vi "Turn To Angle Teleop.vi"(8 "Z Axis":dbl, 9 "PID gains":T1={"proportional gain (Kc)"=0.035, "integral time (Ti, min)"=0.0, "derivative time (Td, min)"=0.0018}, 10 "POV":i16(knob) scale=0.0..360.0, 11 "output range":cluster{"output high":dbl, "output low":dbl}={"output high"=1.0, "output low"=-1.0}) -> (2 "Adjustment Voltage":dbl)   [LabVIEW 2018]
uses:
  <vilib>/addons/control/pid/pid.llb/PID (DBL).vi
  <vilib>/addons/control/pid/NI_PID_pid.lvlib
panel:
  # ".0202"
  # "0"
  # ".0032150"
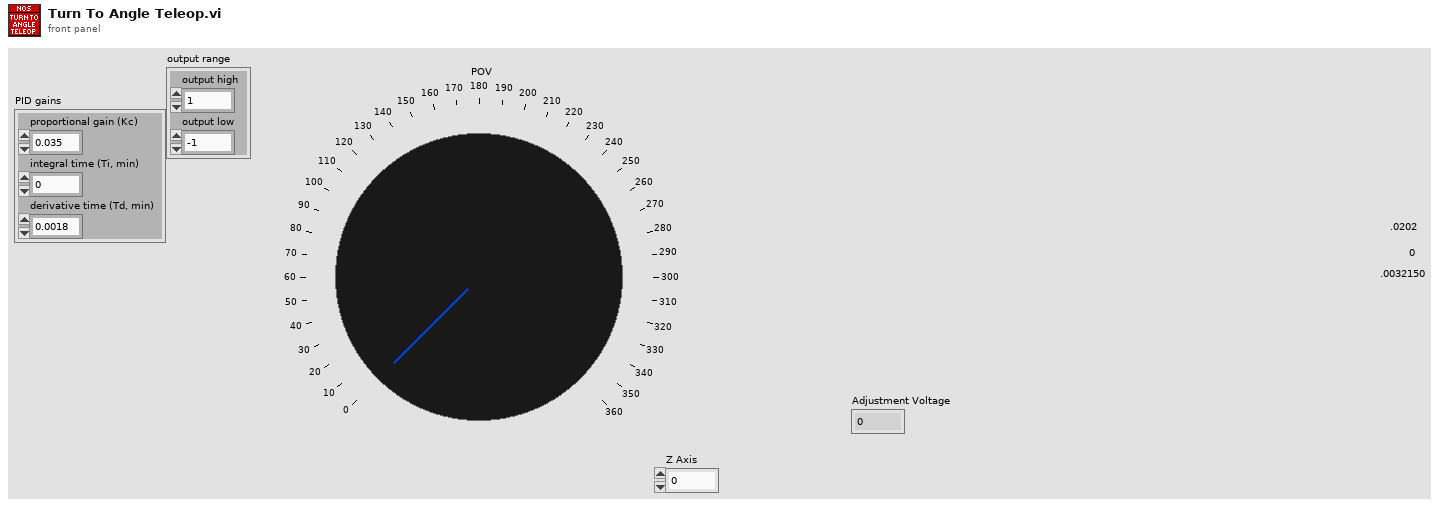
[diagram p1: front panel]
types:
  T1 = cluster{"proportional gain (Kc)":dbl, "integral time (Ti, min)":dbl, "derivative time (Td, min)":dbl}
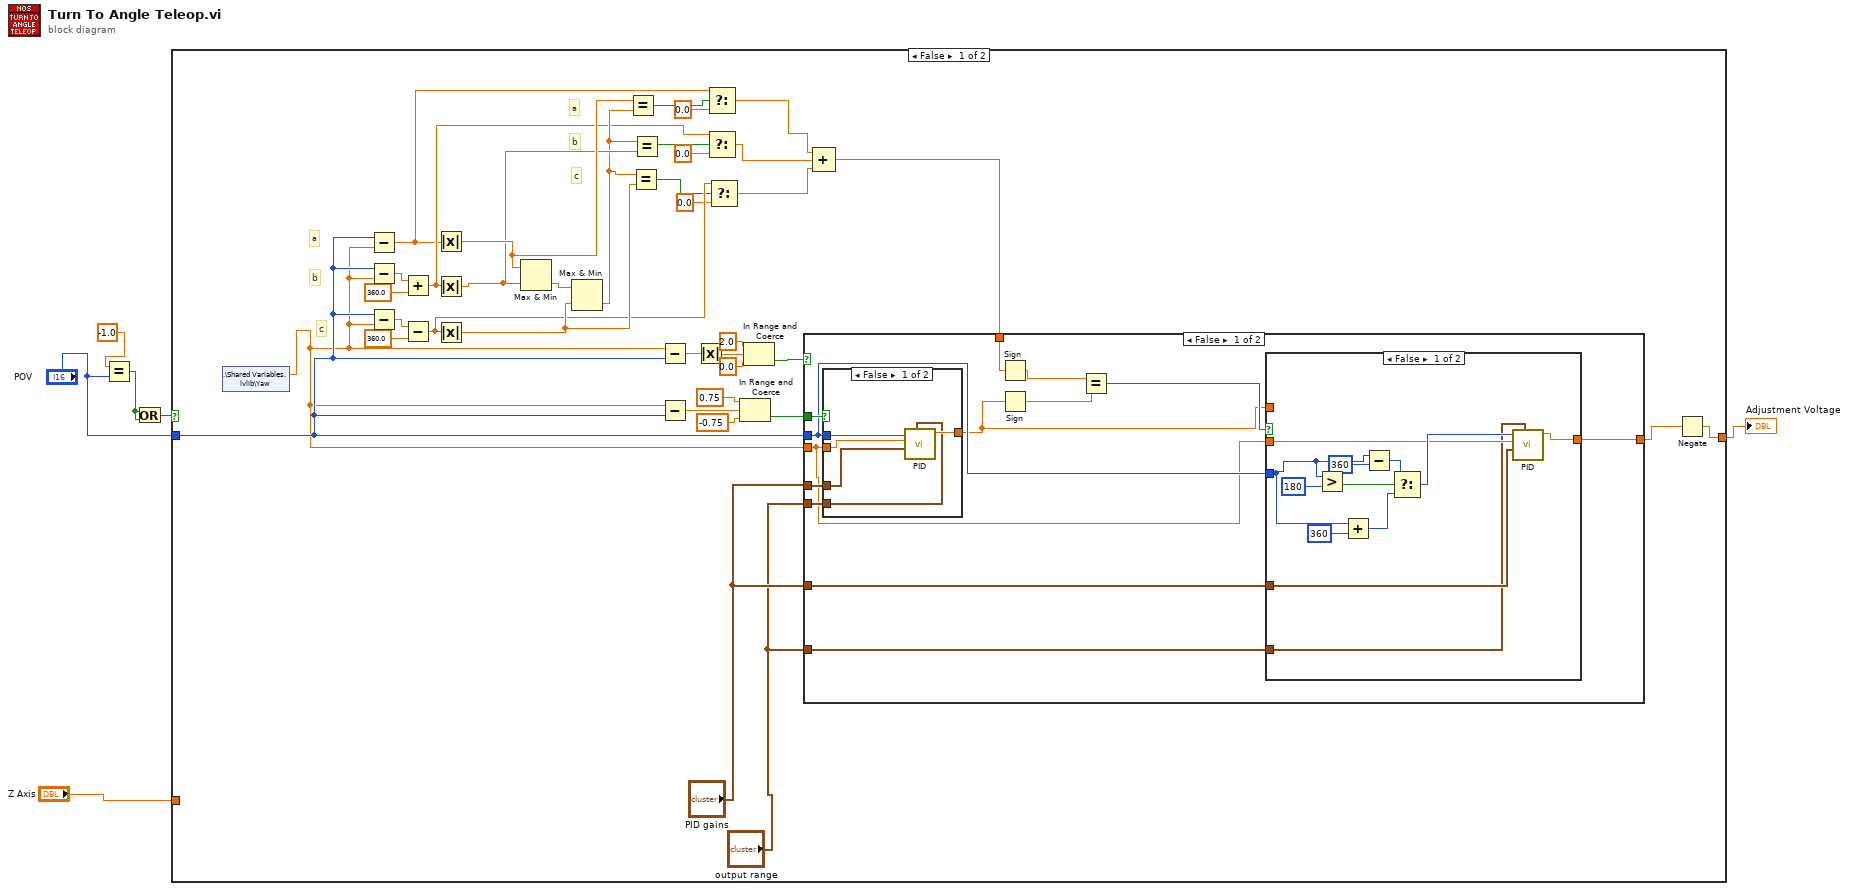
[diagram p0: block diagram]
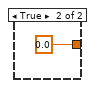
[diagram p3: hidden frame]
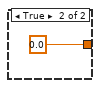
[diagram p4: hidden frame]
diagram:
  n1 = Equal?(x=-1.0, y="POV") -> (x = y?=w1:bool)
  n2 = Or(x=w1, y=w1) -> (x .or. y?=w2:bool)
  n3 = case shown="False" w2 {
    tunnel: "POV" -> [w12 _]
    tunnel: [w13 w77] -> w5
    tunnel: "Z Axis" -> [_ w77]
    frame False {
      # "c"
      # "b"
      # "a"
      # "c"
      # "b"
      # "a"
      n4 = shared-variable ".\\Shared Variables.lvlib\\Yaw"() -> (w7:dbl)  [unwired: 1 in, 1 out]
      n5 = Subtract(x=w12, y=w7) -> (x-y=w23:dbl)
      n6 = Subtract(x=w12, y=w7) -> (x-y=w34:dbl)
      n7 = Subtract(x=w12, y=w7) -> (x-y=w32:dbl)
      n8 = Add(x=w34, y=360.0) -> (x+y=w24:dbl)
      n9 = Subtract(x=w32, y=360.0) -> (x-y=w22:dbl)
      n10 = Absolute Value(x=w23) -> (abs(x)=w29:dbl)
      n11 = Absolute Value(x=w24) -> (abs(x)=w28:dbl)
      n12 = Absolute Value(x=w22) -> (abs(x)=w26:dbl)
      n13 = Max & Min(x=w29, y=w28) -> (min(x,y)=w30:dbl)  [unwired: 1 out]
      n14 = Max & Min(x=w30, y=w26) -> (min(x,y)=w27:dbl)  [unwired: 1 out]
      n15 = Equal?(x=w29, y=w27) -> (x = y?=w21:bool)
      n16 = Equal?(x=w27, y=w26) -> (x = y?=w20:bool)
      n17 = Equal?(x=w27, y=w28) -> (x = y?=w25:bool)
      n18 = Subtract(x=w7, y=w12) -> (x-y=w41:dbl)
      n19 = Subtract(x=w7, y=w12) -> (x-y=w39:dbl)
      n20 = Absolute Value(x=w41) -> (abs(x)=w40:dbl)
      n21 = Select(t=w23, s=w21, f=0.0) -> (s? t:f=w16:dbl)
      n22 = Select(t=w24, s=w25, f=0.0) -> (s? t:f=w15:dbl)
      n23 = Select(t=w22, s=w20, f=0.0) -> (s? t:f=w14:dbl)
      n24 = In Range and Coerce(upper limit=0.75, x=w39, lower limit=-0.75) -> (In Range?=w36:bool)  [unwired: 1 out]
      n25 = In Range and Coerce(upper limit=2.0, x=w40, lower limit=0.0) -> (In Range?=w35:bool)  [unwired: 1 out]
      n26 = Compound Arithmetic op=ADD(w16, w15, w14) -> (w11:dbl)
      n27 = case shown="False" w35 {
        tunnel: w7 -> [w47 _]
        tunnel: w36 -> [w56 _]
        tunnel: w12 -> [w48 _]
        tunnel: "PID gains" -> [w55 _]
        tunnel: "output range" -> [w54 _]
        tunnel: w11 -> [w51 _]
        tunnel: [w50 0.0 ("output")] -> w10
        tunnel: "PID gains" -> [w46 _]
        tunnel: "output range" -> [w45 _]
        frame False {
          n28 = case shown="False" w56 {
            tunnel: w47 -> [w74 _]
            tunnel: w48 -> [w72 _]
            tunnel: [w73 0.0 ("output")] -> w44
            tunnel: w55 -> [w71 _]
            tunnel: w54 -> [w70 _]
            frame False {
              n29 = call-poly <vilib>:"PID.vi"("output range"=w70, "PID gains"=w71, "process variable"=w74, "setpoint"=w72) -> ("output"=w73:dbl)  [unwired: 6 in, 1 out]
            }
            frame True {
            }
          }
          n30 = Sign(1:w51) -> (0:w52:dbl)
          n31 = Sign(1:w44) -> (0:w53:dbl)
          n32 = Equal?(x=w52, y=w53) -> (x = y?=w49:bool)
          n33 = case shown="False" w49 {
            tunnel: [w68 w69] -> w50
            tunnel: w48 -> [w60 _]
            tunnel: w47 -> [w59 _]
            tunnel: w46 -> [w58 _]
            tunnel: w45 -> [w57 _]
            tunnel: w44 -> [_ w69]
            frame False {
              n34 = Greater?(x=w60, y=i16 180) -> (0:w66:bool)
              n35 = Add(x=w60, y=i16 360) -> (x+y=w64:i16)
              n36 = Subtract(x=w60, y=i16 360) -> (x-y=w62:i16)
              n37 = Select(t=w62, s=w66, f=w64) -> (s? t:f=w61:i16)
              n38 = call-poly <vilib>:"PID.vi"("output range"=w57, "PID gains"=w58, "process variable"=w59, "setpoint"=w61) -> ("output"=w68:dbl)  [unwired: 6 in, 1 out]
            }
            frame True {
            }
          }
        }
        frame True {
        }
      }
      n39 = Negate(x=w10) -> (-x=w13:dbl)
    }
    frame True {
    }
  }
  "Adjustment Voltage" <- w5
